vi "airplane__cluster_v2.vi"() -> ()   [LabVIEW 2021]
uses:
  <vilib>/numeric/Random Number (Range) U64.vi
  <vilib>/numeric/sub_Random U32.vi
panel:
  out "Messages for passengers":string="fly"
  out "braking speed":dbl(knob) scale=0.0..2000.0
  out "braking high":u8(slide) scale=0.0..100.0
  out "now speed":dbl(knob) scale=0.0..2000.0
  out "fuel":dbl(slide) scale=0.0..3000.0
  out "fuel":dbl
  out "start fuel":dbl
  out "flight instructions":string="let's go!"
  out "high":u8(slide) scale=0.0..100.0
  out "braking high":dbl
  out "braking speed":dbl
  out "speed now":dbl
  out "high now":dbl
  out "airplane position":cluster{dbl[], dbl[]}(graph)
  out "now position y":dbl
  out "now position x":dbl
  in  "airplane":T1
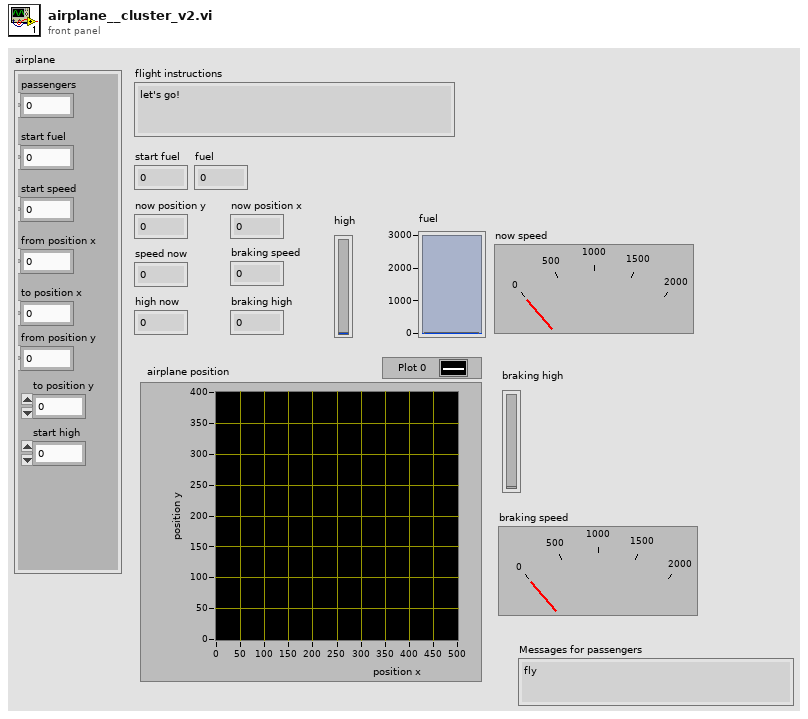
[diagram p1: front panel]
types:
  T1 = cluster{"passengers":dbl, "start fuel":dbl, "start speed":dbl, "from position x":dbl, "to position x":dbl, "start high":dbl, "to position y":dbl, "from position y":dbl}
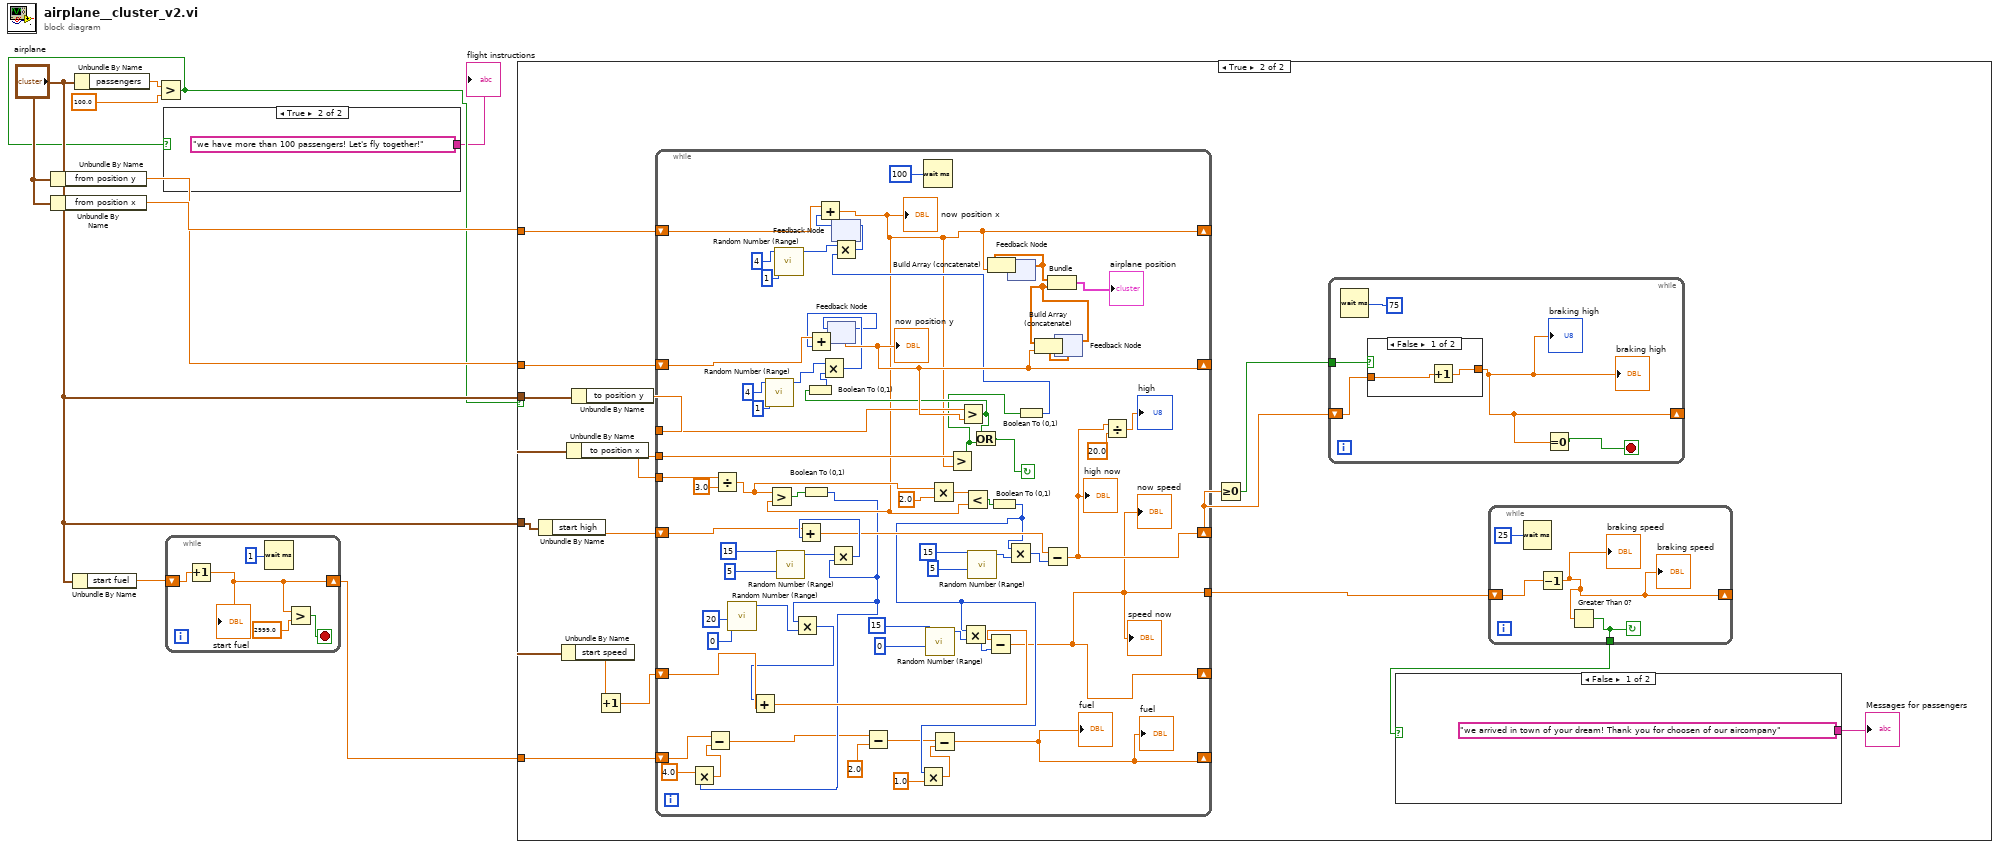
[diagram p0: block diagram]
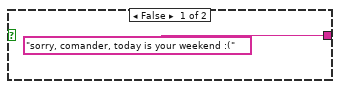
[diagram p2: hidden frame]
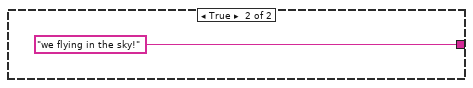
[diagram p4: hidden frame]
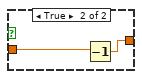
[diagram p5: hidden frame]
diagram:
  n1 = Unbundle By Name("airplane") -> ("from position y"=w6:dbl)
  n2 = Unbundle By Name("airplane") -> ("from position x"=w7:dbl)
  n3 = Unbundle By Name("airplane") -> ("start fuel"=w2:dbl)
  n4 = Unbundle By Name("airplane") -> ("passengers"=w9:dbl)
  n5 = Greater?(x=w9, y=100.0) -> (0:w4:bool)
  n6 = case shown="True" w4 {
    tunnel: ["sorry, comander, today is your weekend :(" "we have more than 100 passengers! Let's fly together!"] -> w3
    frame False {
    }
    frame True {
    }
  }
  "flight instructions" <- w3
  n7 = while {
    shift-right: [w13] -> w1
    shift-left: w2 -> [w16]
    stop <- w15 stop-if-true
    n8 = Increment(x=w16) -> (x+1=w13:dbl)
    "start fuel" <- w13
    n9 = Wait (ms)(milliseconds to wait=u32 1) -> ()  [unwired: 1 out]
    n10 = Greater?(x=w13, y=2999.0) -> (0:w15:bool)
  }
  n11 = case shown="True" w4 {
    tunnel: w7 -> [_ w31]
    tunnel: w6 -> [_ w30]
    tunnel: "airplane" -> [_ w22]
    tunnel: "airplane" -> [_ w21]
    tunnel: w1 -> [_ w19]
    frame False {
    }
    frame True {
      n12 = Unbundle By Name(w21) -> ("start high"=w20:dbl)
      n13 = Unbundle By Name(w22) -> ("start speed"=w27:dbl)
      n14 = Unbundle By Name(w22) -> ("to position x"=w28:dbl)
      n15 = Unbundle By Name(w22) -> ("to position y"=w29:dbl)
      n16 = Increment(x=w27) -> (x+1=w26:dbl)
      n17 = while {
        shift-right: [w75] -> _
        shift-left: w31 -> [w112]
        shift-right: [w103] -> _
        shift-left: w30 -> [w109]
        tunnel: w29 -> [w102]
        tunnel: w28 -> [w101]
        tunnel: w28 -> [w89]
        shift-right: [w60] -> w23
        shift-left: w20 -> [w82]
        shift-right: [w47] -> _
        shift-left: w26 -> [w71]
        tunnel: [w47] -> w25
        shift-right: [w48] -> _
        shift-left: w19 -> [w58]
        stop <- w100 continue-if-true
        n18 = Divide(x=w89, y=3.0) -> (x/y=w81:dbl)
        n19 = call-poly <vilib>:"Random Number (Range).vi"("lower bound (0)"=u64 0, "upper bound (100)"=u64 20) -> ("number"=w68:u64)  [unwired: 9 in]
        n20 = call-poly <vilib>:"Random Number (Range).vi"("lower bound (0)"=u64 1, "upper bound (100)"=u64 4) -> ("number"=w97:u64)  [unwired: 9 in]
        n21 = call-poly <vilib>:"Random Number (Range).vi"("lower bound (0)"=u64 1, "upper bound (100)"=u64 4) -> ("number"=w92:u64)  [unwired: 9 in]
        n22 = call-poly <vilib>:"Random Number (Range).vi"("lower bound (0)"=u64 5, "upper bound (100)"=u64 15) -> ("number"=w84:u64)  [unwired: 9 in]
        n23 = feedback #1() -> (w95:u64)  [unwired: 1 in]
        n24 = Add(x=w109, y=w95) -> (x+y=w103:dbl)
        "now position y" <- w103
        n25 = feedback #2() -> (w90:u64)  [unwired: 1 in]
        n26 = Add(x=w112, y=w90) -> (x+y=w75:dbl)
        "now position x" <- w75
        n27 = Greater?(x=w81, y=w75) -> (0:w85:bool)
        n28 = Boolean To (0,1)(Boolean=w85) -> (0, 1=w56:i16)
        n29 = Multiply(x=4.0 ("y"), y=w56) -> (x*y=w55:dbl)
        n30 = Subtract(x=w58, y=w55) -> (x-y=w53:dbl)
        n31 = Multiply(x=w56, y=w68) -> (x*y=w67:u64)
        n32 = Add(x=w67, y=w71) -> (x+y=w63:dbl)
        n33 = Multiply(x=w84, y=w56) -> (x*y=w83:u64)
        n34 = Add(x=w82, y=w83) -> (x+y=w73:dbl)
        n35 = Subtract(x=w53, y=2.0 ("x")) -> (x-y=w49:dbl)
        n36 = Wait (ms)(milliseconds to wait=u32 100) -> ()  [unwired: 1 out]
        n37 = call-poly <vilib>:"Random Number (Range).vi"("lower bound (0)"=u64 0, "upper bound (100)"=u64 15) -> ("number"=w64:u64)  [unwired: 9 in]
        n38 = Multiply(x=w81, y=2.0) -> (x*y=w76:dbl)
        n39 = Greater?(x=w101, y=w75) -> (0:w94:bool)
        n40 = Greater?(x=w102, y=w103) -> (0:w99:bool)
        n41 = Boolean To (0,1)(Boolean=w99) -> (0, 1=w98:i16)
        n42 = Multiply(x=w97, y=w98) -> (x*y=w96:u64)
        n43 = feedback-in #1(w96) -> ()
        n44 = Less?(x=w76, y=w75) -> (x < y?=w72:bool)
        n45 = call-poly <vilib>:"Random Number (Range).vi"("lower bound (0)"=u64 5, "upper bound (100)"=u64 15) -> ("number"=w77:u64)  [unwired: 9 in]
        n46 = Or(x=w99, y=w94) -> (x .or. y?=w100:bool)
        n47 = Boolean To (0,1)(Boolean=w72) -> (0, 1=w51:i16)
        n48 = Multiply(x=w51, y=1.0) -> (x*y=w50:dbl)
        n49 = Subtract(x=w49, y=w50) -> (x-y=w48:dbl)
        "fuel" <- w48
        "fuel" <- w48
        n50 = Multiply(x=w51, y=w64) -> (x*y=w62:u64)
        n51 = Subtract(x=w63, y=w62) -> (x-y=w47:dbl)
        "speed now" <- w47
        "now speed" <- w47
        n52 = Multiply(x=w51, y=w77) -> (x*y=w74:u64)
        n53 = feedback #3() -> (w104:dbl[])  [unwired: 1 in]
        n54 = Build Array (concatenate)(w104, w75) -> (w105:dbl[])
        n55 = feedback-in #3(w105) -> ()
        n56 = Boolean To (0,1)(Boolean=w94) -> (0, 1=w93:i16)
        n57 = Multiply(x=w92, y=w93) -> (x*y=w91:u64)
        n58 = feedback-in #2(w91) -> ()
        n59 = Subtract(x=w73, y=w74) -> (x-y=w60:dbl)
        "high now" <- w60
        n60 = feedback #4() -> (w106:dbl[])  [unwired: 1 in]
        n61 = Build Array (concatenate)(w106, w103) -> (w107:dbl[])
        n62 = Bundle(w104, w106) -> (→"airplane position":cluster{dbl[], dbl[]})  [unwired: 1 in]
        n63 = feedback-in #4(w107) -> ()
        n64 = Divide(x=w60, y=20.0) -> (x/y=→"high":dbl)
      }
      n65 = Greater Or Equal To 0?(x=w23) -> (x >= 0?=w24:bool)
      n66 = while {
        shift-right: [w34] -> _
        shift-left: w23 -> [w36]
        tunnel: w24 -> [w37]
        stop <- w35 stop-if-true
        n67 = Wait (ms)(milliseconds to wait=u32 75) -> ()  [unwired: 1 out]
        n68 = case shown="False" w37 {
          tunnel: w36 -> [w39 w42]
          tunnel: [w40 w41] -> w34
          frame False {
            n69 = Increment(x=w39) -> (x+1=w40:dbl)
          }
          frame True {
            n70 = Decrement(x=w42) -> (x-1=w41:dbl)
          }
        }
        "braking high" <- w34
        "braking high" <- w34
        n71 = Equal To 0?(x=w34) -> (x = 0?=w35:bool)
      }
      n72 = while {
        shift-right: [w44] -> _
        shift-left: w25 -> [w45]
        tunnel: [w43] -> w18
        stop <- w43 continue-if-true
        n73 = Wait (ms)(milliseconds to wait=u32 25) -> ()  [unwired: 1 out]
        n74 = Decrement(x=w45) -> (x-1=w44:dbl)
        "braking speed" <- w44
        "braking speed" <- w44
        n75 = Greater Than 0?(x=w44) -> (x > 0?=w43:bool)
      }
      n76 = case shown="False" w18 {
        tunnel: ["we arrived in town of your dream! Thank you for choosen of our aircompany" "we flying in the sky!"] -> w17
        frame False {
        }
        frame True {
        }
      }
      "Messages for passengers" <- w17
    }
  }
